vi "Update Run Instance Parameters.vi"(8 "error in (no error)":errorcluster, 10 "Parameters":string[][](array[string]), 11 "Optimiser Cell in":refnum<class "Optimiser Cell.lvclass">) -> (0 "error out":errorcluster, 3 "Optimiser Cell out":refnum<class "Optimiser Cell.lvclass">)   [LabVIEW 2020, in "CIRCUS_uServices.lvlib" / "Run Utilities.lvlib" / "Optimiser Cell.lvclass"]
uses:
  Optimiser Cell.lvclass
  Optimiser Cell.lvclass/Optimiser Cell.ctl
  TALOS/TALOS_PPL.lvlibp
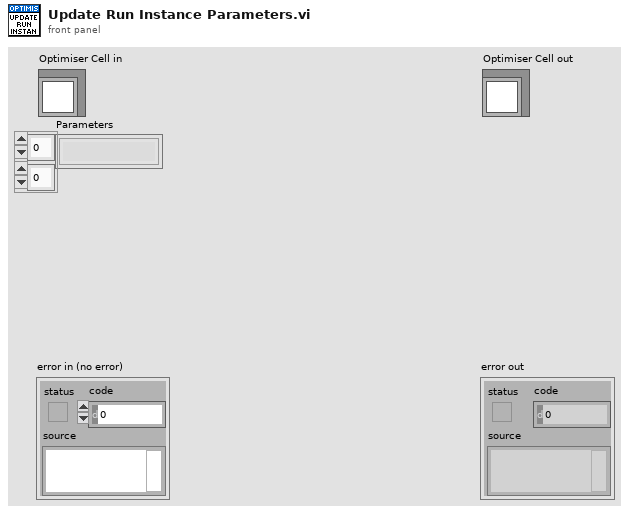
[diagram p1: front panel]
types:
  T1 = typedef "CIRCUS_uServices.lvlib/Run Utilities.lvlib/Optimiser Cell.lvclass/Optimise parameter - numeric.ctl" = cluster{"Name":string, "Start value":dbl, "From":dbl, "To":dbl, "dtype":enum16{"INT", "DBL"}}
  T2 = typedef "CIRCUS_uServices.lvlib/Run Utilities.lvlib/Optimiser Cell.lvclass/Optimise parameter - string.ctl" = cluster{"Name":string, "Start value":string, "Options":string[]}
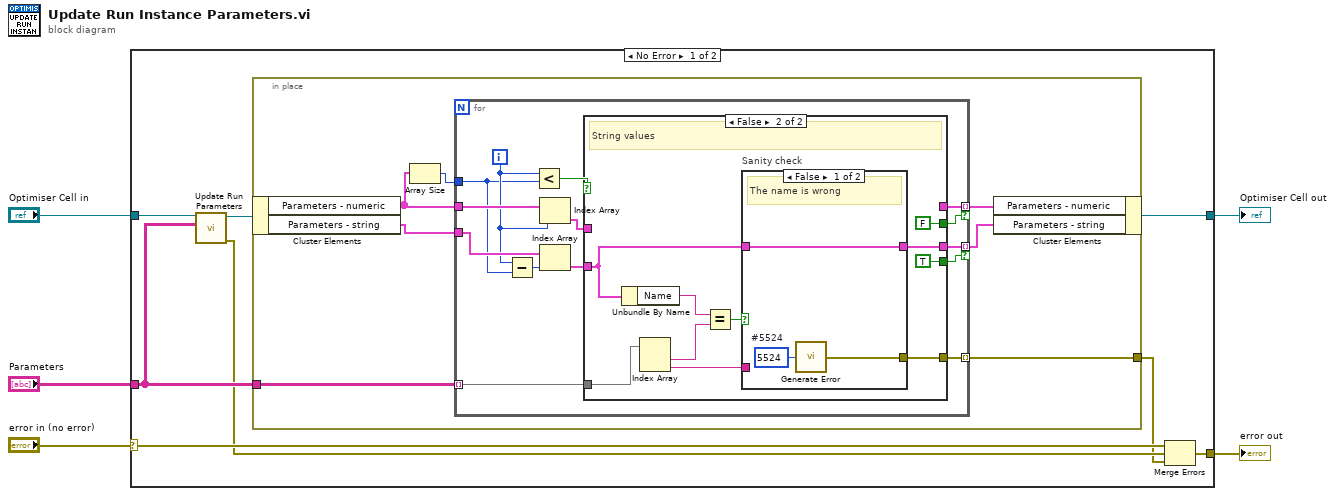
[diagram p0: block diagram]
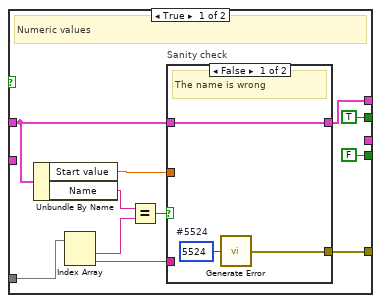
[diagram p2: hidden frame]
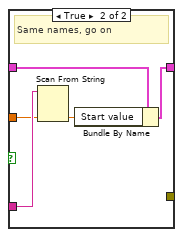
[diagram p3: hidden frame]
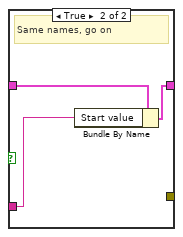
[diagram p4: hidden frame]
diagram:
  n1 = case shown="No Error" "error in (no error)" {
    selector: "error in (no error)" -> [w13 w71]
    tunnel: [w6 w71] -> w4
    tunnel: [w12 w70] -> w2
    tunnel: "Optimiser Cell in" -> [w11 w70]
    tunnel: "Parameters" -> [w9 _]
    frame No Error {
      n2 = call-dynamic "Update Run Parameters.vi"("Parameters"=w9, "Optimiser Cell in"=w11) -> ("error out"=w8:errorcluster, "Optimiser Cell out"=w10:refnum<class "Optimiser Cell.lvclass">)  [unwired: 8 in]
      n3 = in-place {
        in-place-border: w9 -> [w20]
        in-place-border: [w14] -> w7
        n4 = in-place-cluster #1(w10) -> ("Parameters - numeric"=w19:T1[], "Parameters - string"=w18:T2[])
        n5 = Array Size(array=w19) -> (size(s)=w17:i32)
        n6 = for {
          tunnel: w20 -> [w33] mode=indexing
          tunnel: w19 -> [w32]
          tunnel: w18 -> [w30]
          tunnel: w17 -> [w28]
          tunnel: [w25] -> w16 mode=indexing if=w22
          tunnel: [w24] -> w14 mode=indexing
          tunnel: [w23] -> w15 mode=indexing if=w21
          i -> [w29]
          n7 = Subtract(x=w29, y=w28) -> (x-y=w27:i32)
          n8 = Less?(x=w29, y=w28) -> (x < y?=w34:bool)
          n9 = Index Array(array=w32, index=w29) -> (element=w31:T1)
          n10 = Index Array(array=w30, index=w27) -> (element=w26:T2)
          n11 = case shown="False" w34 {
            tunnel: w31 -> [w40 _]
            tunnel: w33 -> [w45 w63]
            tunnel: w26 -> [_ w57]
            tunnel: [w39 _] -> w25
            tunnel: [w38 w58] -> w24
            tunnel: [_ w56] -> w23
            tunnel: [TRUE FALSE] -> w22
            tunnel: [FALSE TRUE] -> w21
            frame True {
              # "Numeric values"
              n12 = Unbundle By Name(w40) -> ("Start value"=w37:dbl, "Name"=w44:string)
              n13 = Index Array(array=w45) -> (element #1=w43:string, element #2=w41:string)  [unwired: 2 in]
              n14 = Equal?(x=w44, y=w43) -> (x = y?=w42:bool)
              n15 = case "Sanity check" shown="False" w42 {
                tunnel: w41 -> [_ w53]
                tunnel: w40 -> [w48 w51]
                tunnel: [w48 w50] -> w39
                tunnel: [w46 _] -> w38
                tunnel: w37 -> [_ w49]
                frame False {
                  w47 = 5524  # #5524
                  # "The name is wrong"
                  n16 = call "Generate Error.vi"("Error Code"=w47) -> ("error out"=w46:errorcluster)  [unwired: 6 in]
                }
                frame True {
                  # "Same names, go on"
                  n17 = Scan From String(input string=w53, default 1=w49) -> (output 1=w52:dbl)  [unwired: 3 in, 3 out]
                  n18 = Bundle By Name(cluster=w51, "Start value"=w52) -> (w50:T1)
                }
              }
            }
            frame False {
              # "String values"
              n19 = Unbundle By Name(w57) -> ("Name"=w62:string)
              n20 = Index Array(array=w63) -> (element #1=w61:string, element #2=w59:string)  [unwired: 2 in]
              n21 = Equal?(x=w62, y=w61) -> (x = y?=w60:bool)
              n22 = case "Sanity check" shown="False" w60 {
                tunnel: w59 -> [_ w67]
                tunnel: w57 -> [w66 w69]
                tunnel: [w66 w68] -> w56
                tunnel: [w64 _] -> w58
                frame False {
                  w65 = 5524  # #5524
                  # "The name is wrong"
                  n23 = call "Generate Error.vi"("Error Code"=w65) -> ("error out"=w64:errorcluster)  [unwired: 6 in]
                }
                frame True {
                  # "Same names, go on"
                  n24 = Bundle By Name(cluster=w69, "Start value"=w67) -> (w68:T2)
                }
              }
            }
          }
        }
        n25 = in-place-cluster #1("Parameters - numeric"=w16, "Parameters - string"=w15) -> (w12:refnum<class "Optimiser Cell.lvclass">)
      }
      n26 = Merge Errors(w13, w8, w7) -> (w6:errorcluster)
    }
    frame Error {
    }
  }
  "error out" <- w4
  "Optimiser Cell out" <- w2
